vi "Calling DLL.vi"() -> ()   [LabVIEW 2021]
panel:
  out "a+b":dbl
  in  "b":dbl
  in  "a":dbl
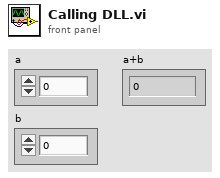
[diagram p1: front panel]
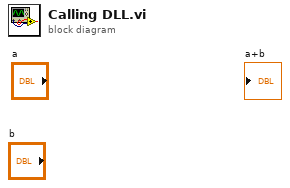
[diagram p0: block diagram]
diagram:
